vi "三态LED.vi"(4 "error in":errorcluster caption="错误输入（无错误）", 5 "State":T1, 7 "Ctl引用句柄":refnum<vi>) -> (0 "error out":errorcluster caption="错误输出", 3 "Ctl引用句柄输出":refnum<vi>)   [LabVIEW 2013]
uses:
  Ctl/LEDState.ctl
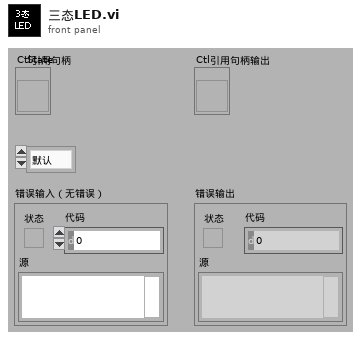
[diagram p1: front panel]
types:
  T1 = typedef "LEDState.ctl" = enum16{"默认", "闪烁", "停止闪烁", "真", "假"}
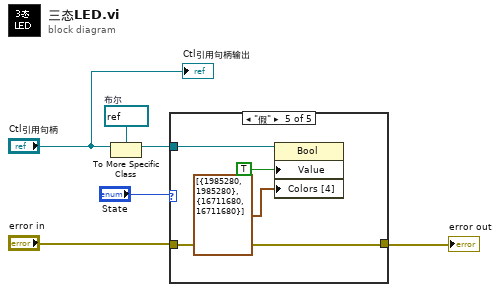
[diagram p0: block diagram]
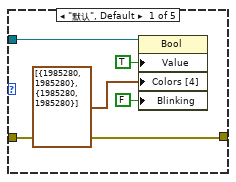
[diagram p2: hidden frame]
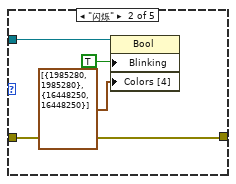
[diagram p3: hidden frame]
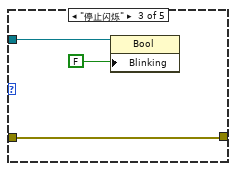
[diagram p4: hidden frame]
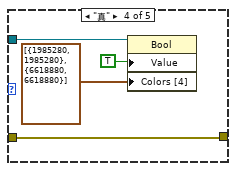
[diagram p5: hidden frame]
diagram:
  w5 = refnum<vi> refnum  # 布尔
  n1 = To More Specific Class(target class=w5, reference="Ctl引用句柄") -> (specific class reference=w4:refnum<vi>)  [unwired: 1 in, 1 out]
  n2 = case shown="\"假\"" "State" {
    tunnel: w4 -> [w10 w14 w17 w20 w24]
    tunnel: "error in" -> [w9 w13 w16 w19 w23]
    tunnel: [w9 w13 w16 w19 w23] -> w2
    frame "默认", Default {
      n3 = property on="属性节点" class="Bool"(reference=w10, "Value"=TRUE ("Boolean"), "Colors [4]"=cluster{u32, u32}[] [{1985280, 1985280}, {1985280, 1985280}], "Blinking"=FALSE ("闪烁")) -> ()  [unwired: 1 in, 2 out]
    }
    frame "闪烁" {
      n4 = property on="属性节点" class="Bool"(reference=w14, "Blinking"=TRUE ("Boolean"), "Colors [4]"=cluster{u32, u32}[] [{1985280, 1985280}, {16448250, 16448250}]) -> ()  [unwired: 1 in, 2 out]
    }
    frame "停止闪烁" {
      n5 = property on="属性节点" class="Bool"(reference=w17, "Blinking"=FALSE ("Boolean")) -> ()  [unwired: 1 in, 2 out]
    }
    frame "真" {
      n6 = property on="属性节点" class="Bool"(reference=w20, "Value"=TRUE ("Boolean"), "Colors [4]"=cluster{u32, u32}[] [{1985280, 1985280}, {6618880, 6618880}]) -> ()  [unwired: 1 in, 2 out]
    }
    frame "假" {
      n7 = property on="属性节点" class="Bool"(reference=w24, "Value"=TRUE ("Boolean"), "Colors [4]"=cluster{u32, u32}[] [{1985280, 1985280}, {16711680, 16711680}]) -> ()  [unwired: 1 in, 2 out]
    }
  }
  "error out" <- w2
  "Ctl引用句柄输出" <- "Ctl引用句柄"
